vi "Write AISAS check.vi"(8 "error in (no error)":errorcluster, 10 "AISAS check":bool=TRUE, 11 "AISAS Mech in":refnum<class "AISAS Mech.lvclass">) -> (0 "error out":errorcluster, 3 "AISAS Mech out":refnum<class "AISAS Mech.lvclass">)   [LabVIEW 2014, in "AISAS Mech.lvclass"]
uses:
  AISAS Mech.lvclass
  AISAS Mech.lvclass/AISAS Mech.ctl
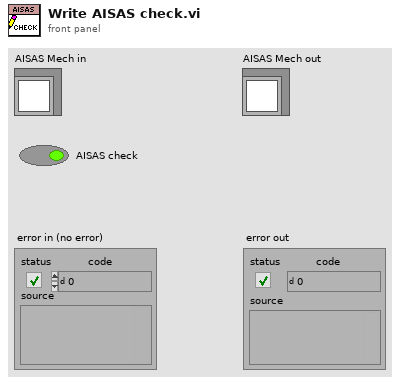
[diagram p1: front panel]
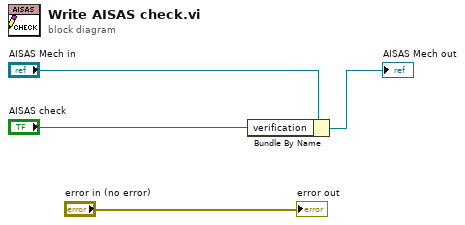
[diagram p0: block diagram]
diagram:
  n1 = Bundle By Name(cluster="AISAS Mech in", "verification"="AISAS check") -> (→"AISAS Mech out":refnum<class "AISAS Mech.lvclass">)
  "error out" <- "error in (no error)"
